vi "displayRejectedCommand.vi"(10 "viewThisComponent":refnum<class "ViewThisComponent.lvclass">) -> ()   [LabVIEW 2015, in "EXAViewElements.lvlib"]
doc: "Displays an indicator element."
uses:
  EXAViewElements.lvlib
  ViewThisComponent/ViewThisComponent.lvclass
  Typedefs/StateValue.ctl
  Typedefs/EXATypedefs.lvlib
  ComponentTemplateCore/ComponentModel/ComponentModel/View/View.lvclass
panel:
  out "Rejected Command":string
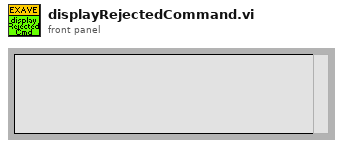
[diagram p1: front panel]
types:
  T1 = typedef "EXATypedefs.lvlib/PubDataEvents.ctl" = cluster{"DetailedState":refnum<user-event>, "ErrorCode":refnum<user-event>, "Heartbeat":refnum<user-event>, "LoopTime_ms":refnum<user-event>, "LoopTimeOutOfRange":refnum<user-event>, "RejectedCommand":refnum<user-event>, "SummaryState":refnum<user-event>, "Timestamp":refnum<user-event>}
  T2 = typedef "EXATypedefs.lvlib/StateValue.ctl" = enum16{"DisabledState", "EnabledState", "FaultState", "OffState", "StandbyState"}
  T3 = typedef "ComponentStateValues.ctl" = enum16{"Off", "Standby", "Enabled", "Disabled", "Fault"}
  T4 = typedef "EXATypedefs.lvlib/CommandValue.ctl" = enum16{"ClearError", "Disable", "Enable", "Exit", "GoToStandby", "OnHeartbeat", "OnIncomingMessagingError", "OnInterrupt", "Start"}
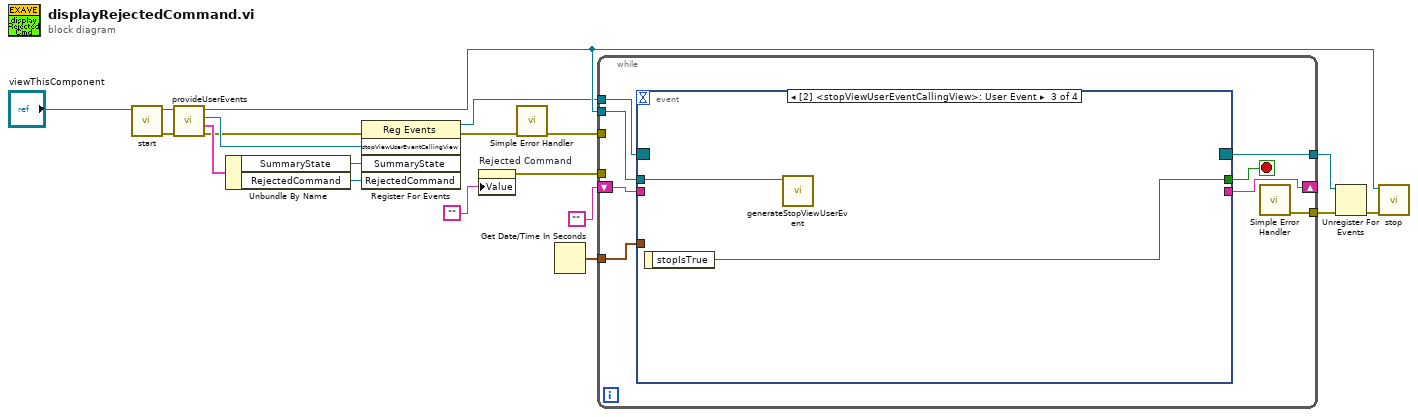
[diagram p0: block diagram]
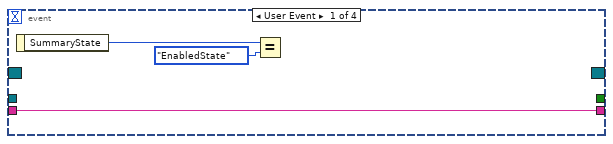
[diagram p2: hidden frame]
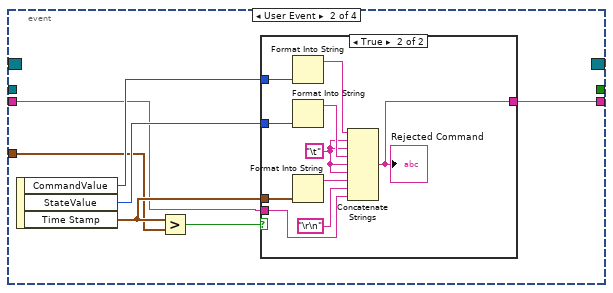
[diagram p3: hidden frame]
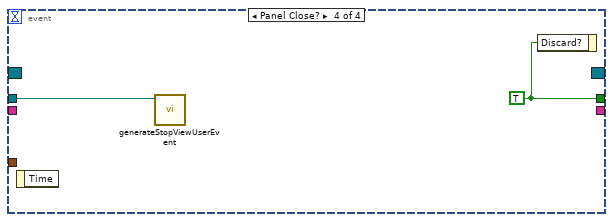
[diagram p5: hidden frame]
diagram:
  n1 = call-dynamic "start.vi"("View in"="viewThisComponent") -> ("error out"=w9:errorcluster, "View out"=w11:refnum<class "ViewThisComponent.lvclass">)  [unwired: 9 in]
  n2 = call "provideUserEvents.vi"("error in (no error)"=w9, "ViewThisComponent in"=w11) -> ("error out"=w12:errorcluster, "pubDataEvents"=w13:T1, "stopViewUserEventCallingView"=w14:refnum<user-event>, "ViewThisComponent out"=w10:refnum<class "ViewThisComponent.lvclass">)  [unwired: 6 in]
  n3 = Unbundle By Name(w13) -> ("SummaryState"=w7:refnum<user-event>, "RejectedCommand"=w6:refnum<user-event>)
  n4 = register-events(error in=w12, w14, w7, w6) -> (reference out=w5:refnum<event-registration>, error out=w4:errorcluster)  [unwired: 1 in]
  n5 = property on="Rejected Command" class="Str"("Value"="") -> (error out=w16:errorcluster)  [unwired: 2 in, 1 out]
  n6 = call <vilib>:"Simple Error Handler.vi"("error in (no error)"=w4) -> ("error out"=w3:errorcluster)  [unwired: 4 in, 4 out]
  n7 = Get Date/Time In Seconds() -> (seconds since 1Jan1904=w18:timestamp)
  n8 = while {
    tunnel: w5 -> [w27]
    tunnel: w10 -> [w26]
    tunnel: [w25] -> w1
    shift-right: [w22] -> _
    shift-left: "" -> [w23]
    tunnel: w18 -> [w21]
    tunnel: w16 -> [_]
    tunnel: [w20] -> w8
    tunnel: w3 -> [_]
    stop <- w24 stop-if-true
    n9 = event shown="[2] <stopViewUserEventCallingView>: User Event" {
      selector: w27 -> [_ _ _ _]
      dyn-events: [_ _ _ _] -> w20
      timeout: _ -> [_ _ _ _]
      tunnel: w26 -> [_ _ w50 w52]
      tunnel: [_ _ w49 w51] -> w24
      tunnel: w23 -> [w30 w33 _ _]
      tunnel: [w30 w32 _ _] -> w22
      tunnel: w21 -> [_ w31 _ _]
      event User Event {
        n10 = event-data() -> ("SummaryState"=w29:T3)  [unwired: 1 in]
        n11 = Equal?(x=w29, y=StateValue."EnabledState" ("StateValue")) -> ()  [unwired: 1 out]
      }
      event User Event {
        n12 = event-data() -> ("CommandValue"=w36:T4, "StateValue"=w35:T2, "Time Stamp"=w34:timestamp)  [unwired: 1 in]
        n13 = Greater?(x=w34, y=w31) -> (0:w37:bool)
        n14 = case shown="True" w37 {
          tunnel: w36 -> [_ w48]
          tunnel: w35 -> [_ w46]
          tunnel: w33 -> [w38 w42]
          tunnel: [w38 w41] -> w32
          tunnel: w34 -> [_ w39]
          frame False {
          }
          frame True {
            w40 = "\t"
            n15 = Format Into String(w48) -> (resulting string=w47:string)  [unwired: 3 in, 1 out]
            n16 = Format Into String(w46) -> (resulting string=w45:string)  [unwired: 3 in, 1 out]
            n17 = Format Into String(w39) -> (resulting string=w44:string)  [unwired: 3 in, 1 out]
            n18 = Concatenate Strings(w47, w40, w40, w45, w40, w40, w44, "\r\n", w42) -> (w41:string)
            "Rejected Command" <- w41
          }
        }
      }
      event User Event {
        n19 = event-data() -> ("stopIsTrue"=w49:bool)  [unwired: 1 in]
        n20 = call "generateStopViewUserEvent.vi"("View in"=w50) -> ()  [unwired: 9 in, 2 out]
      }
      event Panel Close? {
        w51 = TRUE ("Discard?")
        n21 = event-data() -> ()  [unwired: 1 in, 1 out]
        n22 = call "generateStopViewUserEvent.vi"("View in"=w52) -> ()  [unwired: 9 in, 2 out]
        n23 = event-data("Discard?"=w51) -> ()  [unwired: 1 in, 1 out]
      }
    }
    n24 = call <vilib>:"Simple Error Handler.vi"() -> ("error out"=w25:errorcluster)  [unwired: 5 in, 4 out]
  }
  n25 = Unregister For Events(event registration refnum=w8, error in=w1) -> (error out=w2:errorcluster)
  n26 = call-dynamic "stop.vi"("error in (no error)"=w2, "View in"=w10) -> ()  [unwired: 8 in, 2 out]
